vi "Send_B_Status.vi"(8 "error in (no error)":errorcluster, 10 "Status":string, 11 "B_Actor in":refnum<class "B_Actor.lvclass">) -> (0 "error out":errorcluster, 3 "B_Actor out":refnum<class "B_Actor.lvclass">)   [LabVIEW 2025, in "B_Actor.lvlib" / "B_Actor.lvclass"]
uses:
  B_Actor.lvclass
  B_Actor.lvclass/B_Actor.ctl
  C:/Program Files (x86)/National Instruments/LabVIEW 2025/vi.lib/ActorFramework/Actor/Actor.lvclass
  C:/Users/halstead_rideriver/Documents/Labview_Practice/Tasks_Actor/B_Actor/B_Actor.lvclass
  <vilib>/ActorFramework/Actor/Actor.lvclass
  B_Actor Messages/B_msg Msg/B_msg Msg.lvclass
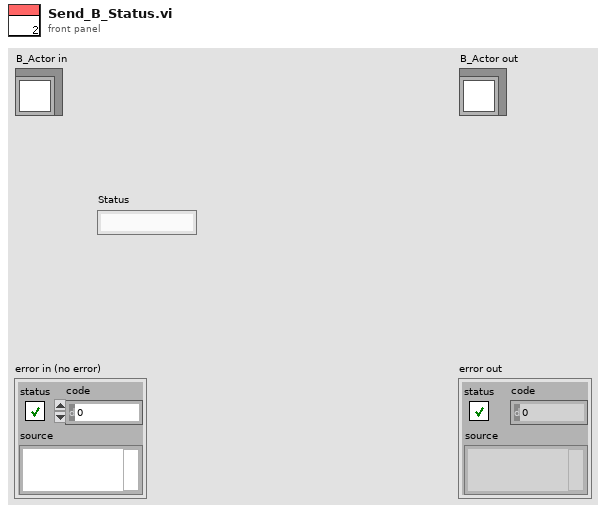
[diagram p1: front panel]
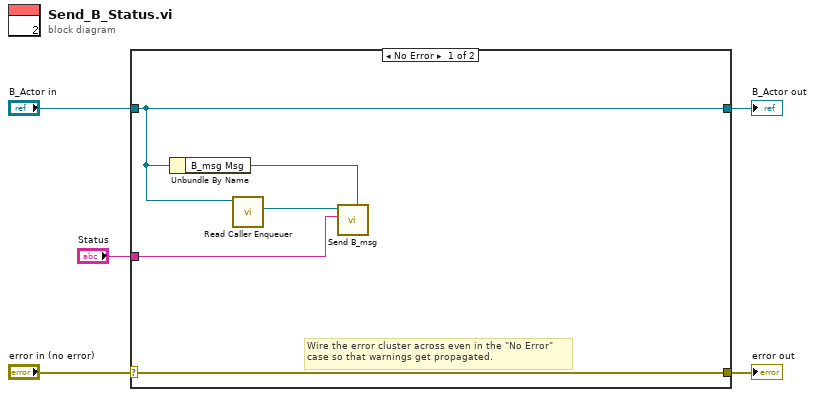
[diagram p0: block diagram]
diagram:
  n1 = case shown="No Error" "error in (no error)" {
    selector: "error in (no error)" -> [w10 w12]
    tunnel: [w10 w12] -> w4
    tunnel: [w9 w11] -> w2
    tunnel: "B_Actor in" -> [w9 w11]
    tunnel: "Status" -> [w6 _]
    frame No Error {
      # "Wire the error cluster across even in the \"No Error\"\ncase so that warnings get propagated."
      n2 = Unbundle By Name(w9) -> ("B_msg Msg"=w7:refnum<class "B_msg Msg.lvclass">)
      n3 = call <vilib>:"Read Caller Enqueuer.vi"("Actor"=w9) -> ("Caller Enqueuer"=w8:refnum<class "Message Enqueuer.lvclass">)  [unwired: 10 in]
      n4 = call "Send B_msg.vi"("Message Type"=w7, "Status"=w6, "Message Enqueuer"=w8) -> ()  [unwired: 7 in, 2 out]
    }
    frame Error {
    }
  }
  "error out" <- w4
  "B_Actor out" <- w2
